vi "Drive to Target (arc).vi"(0 "X":dbl, 1 "Description":string, 5 "Y":dbl, 7 "Max time":dbl, 11 "Command Info In":T2, 12 "Synchronization":enum16{"Start", "Wait"}(ring)) -> (4 "Outcome":string="foo", 15 "Command Info Out":T2)   [LabVIEW 2015]
doc: "This VI sets the motors to run for a given number of seconds. It optionally synchronizes with the completion of the command."
uses:
  <vilib>/Rock Robotics/WPI/Framework/Command Status Info.ctl
  <vilib>/Rock Robotics/WPI/Framework/Completion Status.ctl
  <vilib>/Rock Robotics/WPI/Framework/Completion Notifier.ctl
  Implementation/Drive Setpoints.ctl
  Implementation/Drive Operations.ctl
panel:
  in  "Position":T1
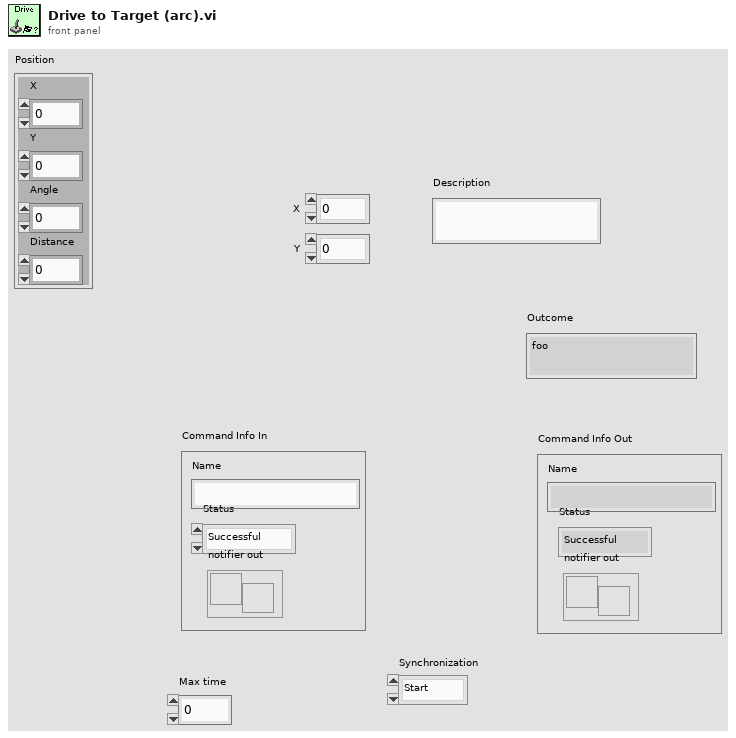
[diagram p1: front panel]
types:
  T1 = cluster{"X":dbl, "Y":dbl, "Angle":dbl, "Distance":dbl}
  T2 = typedef "Command Status Info.ctl" = cluster{"Name":string, "Status":T3, "notifier out":T4}
  T3 = typedef "Completion Status.ctl" = enum16{"Successful", "Aborted", "Incomplete"}
  T4 = typedef "Completion Notifier.ctl" = refnum<notifier>
  T5 = typedef "Drive Setpoints.ctl" = cluster{"Operation":T6, "Left Setpoint":dbl, "Right Setpoint":dbl, "Duration":dbl, "Position":cluster{"X":dbl, "Y":dbl, "Angle":dbl, "Distance":dbl}, "Straight Setpoint":dbl}
  T6 = typedef "Drive Operations.ctl" = enum16{"Reserve", "Read Current", "Immediate", "Turn to Angle", "Drive Straight", "Drive to Target (arc)"}
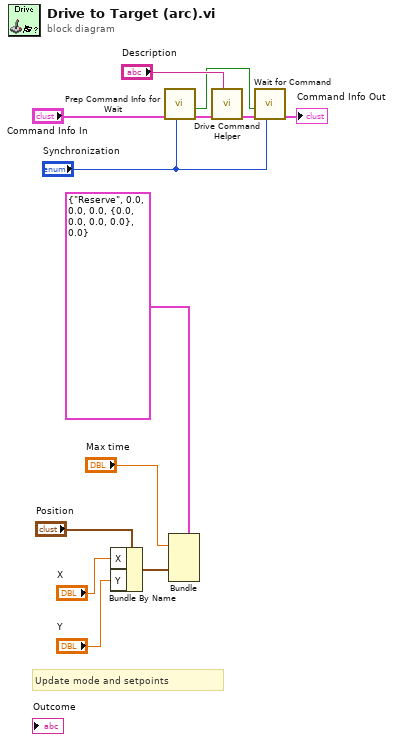
[diagram p0: block diagram]
diagram:
  # "Update mode and setpoints"
  n1 = Bundle By Name(cluster="Position", "X"="X", "Y"="Y") -> (w2:T1)
  n2 = call <vilib>:"Prep Command Info for Wait.vi"("Synchronication"="Synchronization", "Command Info"="Command Info In") -> ("Command Info"=w11:T2, "Allocated"=w12:bool)  [unwired: 8 in]
  n3 = Bundle(cluster=T5 {"Operation"=enum."Reserve", "Left Setpoint"=0.0, "Right Setpoint"=0.0, "Duration"=0.0, "Position"={"X"=0.0, "Y"=0.0, "Angle"=0.0, "Distance"=0.0}, "Straight Setpoint"=0.0} ("SubSystem Data"), "Left Setpoint"="Max time", "Position"=w2) -> ()  [unwired: 4 in, 1 out]
  n4 = call "Drive Command Helper.vi"("Description"="Description", "Command Info In"=w11) -> ("Command Info Out"=w8:T2)  [unwired: 8 in, 1 out]
  n5 = call <vilib>:"Wait for Command.vi"("Synchronication"="Synchronization", "Command Info in"=w8, "Allocated"=w12) -> ("Command Info out"=→"Command Info Out":T2)  [unwired: 8 in]
